vi "AddBlankScore.vi"(7 "P1?":bool, 8 "error in (no error)":errorcluster, 10 "Accessors:Player1Score":i32, 11 "Highscore in":refnum<class "Highscore.lvclass">) -> (0 "error out":errorcluster, 3 "Highscore out":refnum<class "Highscore.lvclass">)   [LabVIEW 2019, in "RT_Game.lvlib" / "Highscore.lvclass"]
uses:
  Highscore.lvclass
  HighscoreEntry.ctl
  Highscore.lvclass/Highscore.ctl
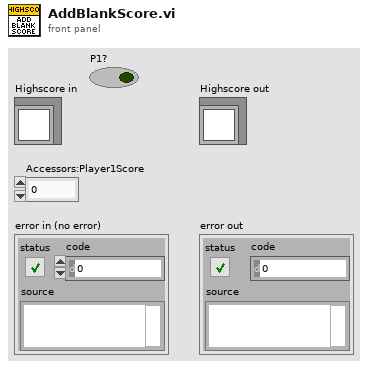
[diagram p1: front panel]
types:
  T1 = typedef "RT_Game.lvlib/Highscore.lvclass/HighscoreEntry.ctl" = cluster{"Name":string, "Score":dbl}
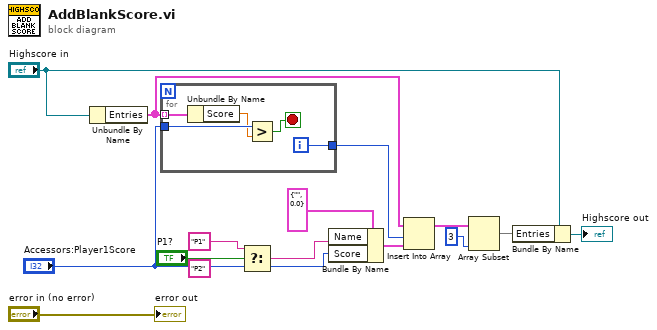
[diagram p0: block diagram]
diagram:
  n1 = Unbundle By Name("Highscore in") -> ("Entries"=w7:T1[])
  n2 = for {
    tunnel: w7 -> [w20] mode=indexing
    tunnel: "Accessors:Player1Score" -> [w19]
    tunnel: [w16] -> w5
    i -> [w16]
    stop <- w17 stop-if-true
    n3 = Unbundle By Name(w20) -> ("Score"=w18:dbl)
    n4 = Greater?(x=w19, y=w18) -> (0:w17:bool)
  }
  n5 = Select(t="P1" ("Name"), s="P1?", f="P2" ("Name")) -> (s? t:f=w2:string)
  n6 = Bundle By Name(cluster=T1 {"Name"="", "Score"=0.0} ("new element/subarray"), "Name"=w2, "Score"="Accessors:Player1Score") -> (w9:T1)
  n7 = Insert Into Array(array=w7, index=w5, new element=w9) -> (w11:T1[])
  n8 = Array Subset(array=w11, length=3) -> (w14:T1[])  [unwired: 1 in]
  n9 = Bundle By Name(cluster="Highscore in", "Entries"=w14) -> (→"Highscore out":refnum<class "Highscore.lvclass">)
  "error out" <- "error in (no error)"
